vi "fgv_file_data.vi"(7 "cmd_file":T1(ring), 8 "err in":errorcluster caption="에러 입력(에러 없음)") -> (0 "error out":errorcluster, 1 "Fail event table":string[][](table), 2 "Strain":waveform(dbl)[](array[waveform]), 3 "Res Acc":waveform(dbl)[](array[waveform]))   [LabVIEW 2016]
panel:
  in  "file path":path
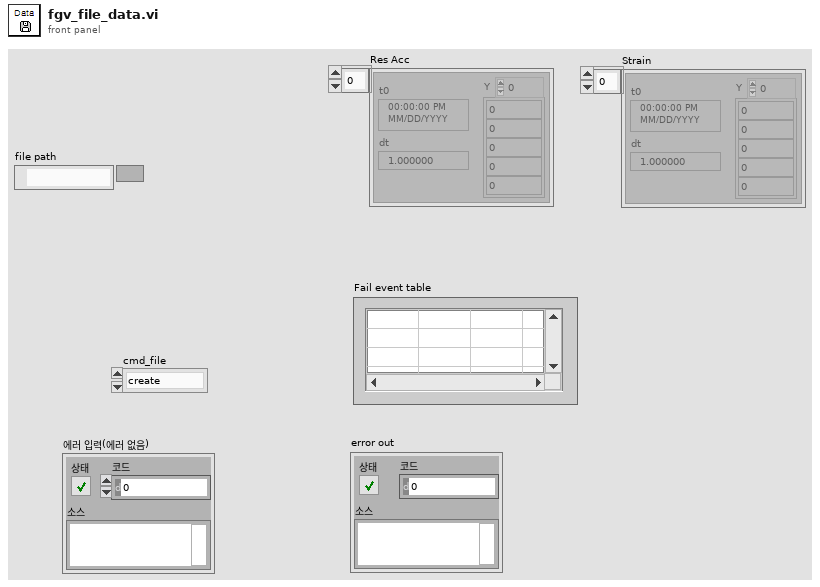
[diagram p1: front panel]
types:
  T1 = enum16{"create", "write_data", "write_event", "read_data", "read_event", "close"}
  T2 = typedef "Total data.ctl" = cluster{"Raw Data":T3, "Resister result data":T4, "Result Table update":cluster{"Num":u32[], "Resister 1~5":u8[][], "Resister 6~10":u8[][], "Resister 11~15":u8[][]}, "Strain Data":cluster{"Strain 1":dbl, "Strain 2":dbl, "Strain 3":dbl, "Strain 4":dbl}, "Acc Result":cluster{"Acc Peak":dbl, "Acc time":dbl, "Acc area":dbl}, "STATUS":cluster{"status":string, "all_fail":bool, "emg":bool, "cycle":u16, "file name":string}, "Speed":dbl, "Acc peak time":dbl, "Max Strain":dbl, "Resistor at peak":cluster{"[0]":dbl, "[1]":dbl, "[2]":dbl, "[3]":dbl, "[4]":dbl, "[5]":dbl, "[6]":dbl, "[7]":dbl, "[8]":dbl, "[9]":dbl, "[10]":dbl, "[11]":dbl, "[12]":dbl, "[13]":dbl, "[14]":dbl}, "Acc peak index":u32, "time":string, "Cycle finish":bool, "Resistor at ini":cluster{"[0]":dbl, "[1]":dbl, "[2]":dbl, "[3]":dbl, "[4]":dbl, "[5]":dbl, "[6]":dbl, "[7]":dbl, "[8]":dbl, "[9]":dbl, "[10]":dbl, "[11]":dbl, "[12]":dbl, "[13]":dbl, "[14]":dbl}}
  T3 = typedef "raw Q data.ctl" = cluster{"Res_data":waveform(dbl)[], "Acc_data":waveform(dbl), "Strain_data":waveform(dbl)[]}
  T4 = typedef "raw data type.ctl" = cluster{"Resistor values":cluster{"[0]":dbl, "[1]":dbl, "[2]":dbl, "[3]":dbl, "[4]":dbl, "[5]":dbl, "[6]":dbl, "[7]":dbl, "[8]":dbl, "[9]":dbl, "[10]":dbl, "[11]":dbl, "[12]":dbl, "[13]":dbl, "[14]":dbl}, "Resistor tables":u8[], "Pass Fails":bool[]}
  T5 = cluster{"Test Information":cluster{"date":string, "custom":string, "oper":string, "package":string, "pkg side":string, "solder":string, "brd side":string, "paste":string, "reflow":string}, "Sensor Set":cluster{"Accelerometer":cluster{"Sensitivity(mV/g)":dbl}, "Strain Guage":cluster{"Ch.":dbl[], "Gage factor":dbl[], "Resistance":dbl[], "Poisson ratio":dbl[]}}, "Resistor Set":cluster{"Criterion Level":dbl, "Res. Set":cluster{"Res. Ch":dbl, "Res. Active":bool, "Res Initial":dbl}[]}, "Test Stop Condition":cluster{"Test cycle":u16, "Fail number in a cycle":u16, "Fail factor":cluster{"Duration":u16, "Fail No.":u16}}, "Acceleration Condition ":cluster{"Shock duration pecent [%]":u16, "Filter cutoff freq":u32}, "Save":cluster{"Save Path":path, "File Name":string}}
  T6 = enum16{"open", "open or create", "create or replace", "create", "open (read-only)"}
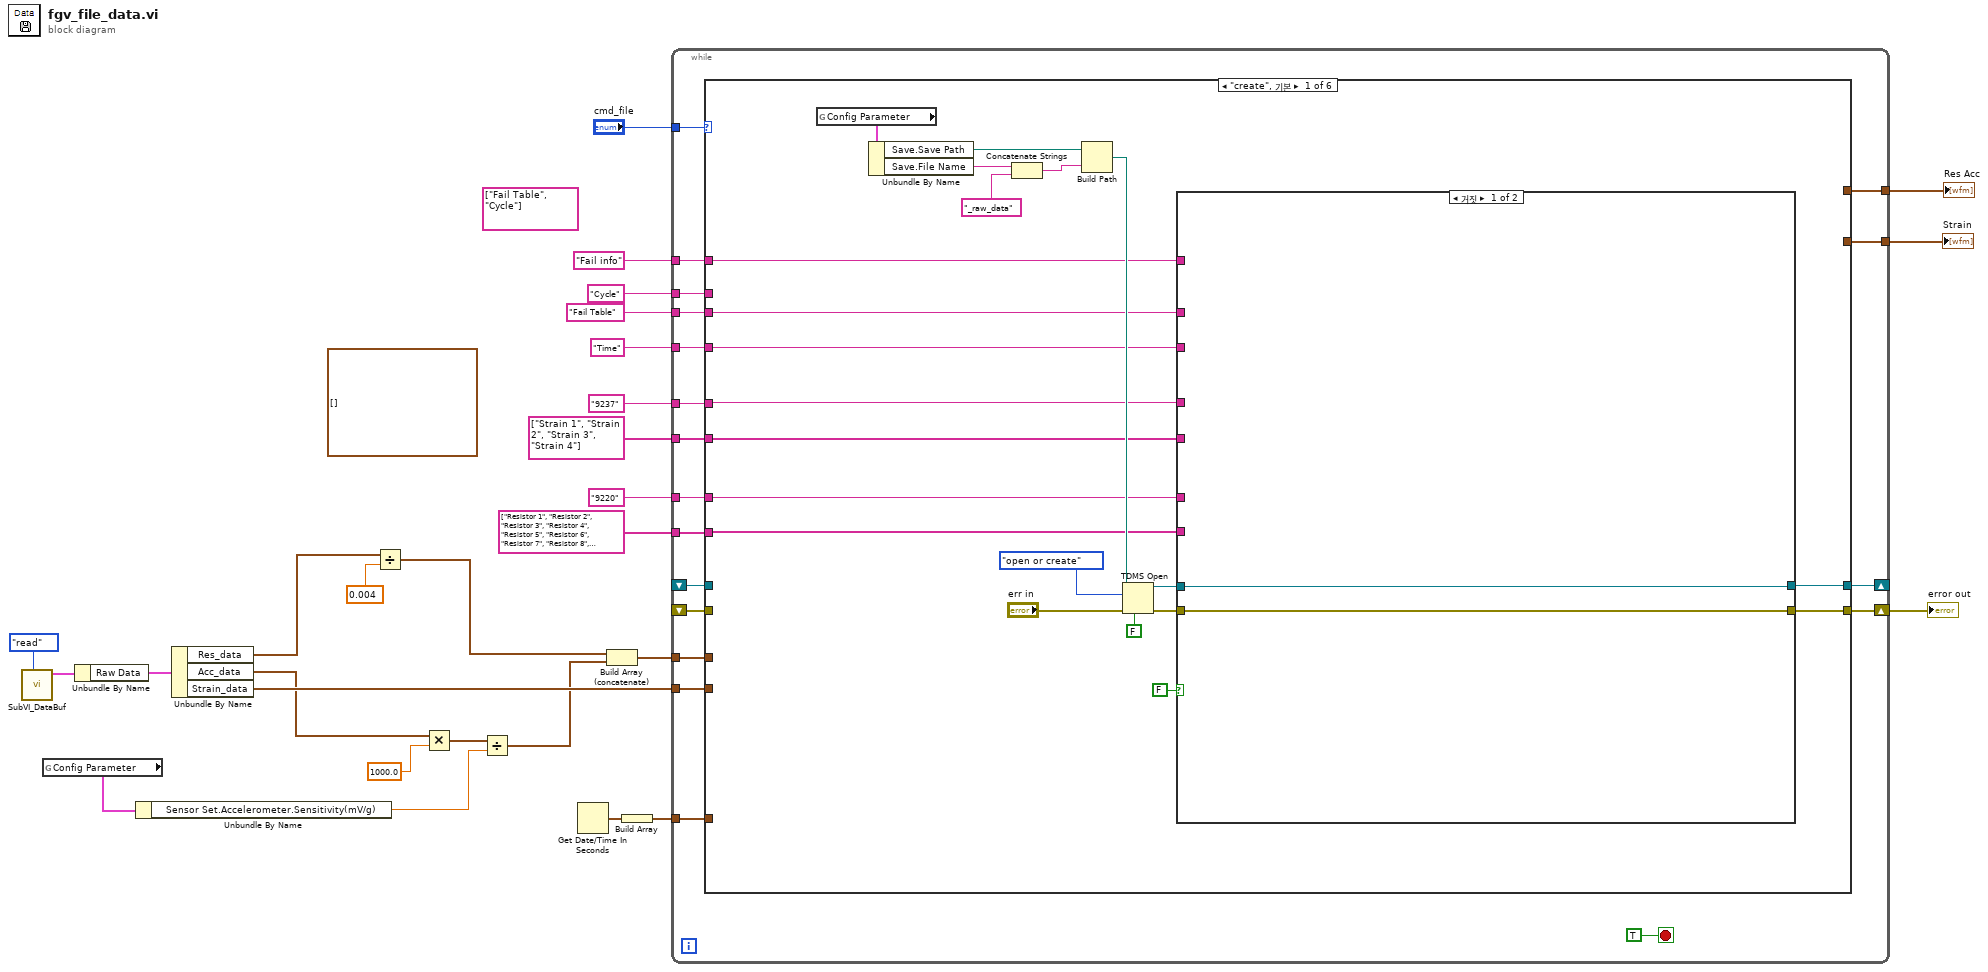
[diagram p0: block diagram]
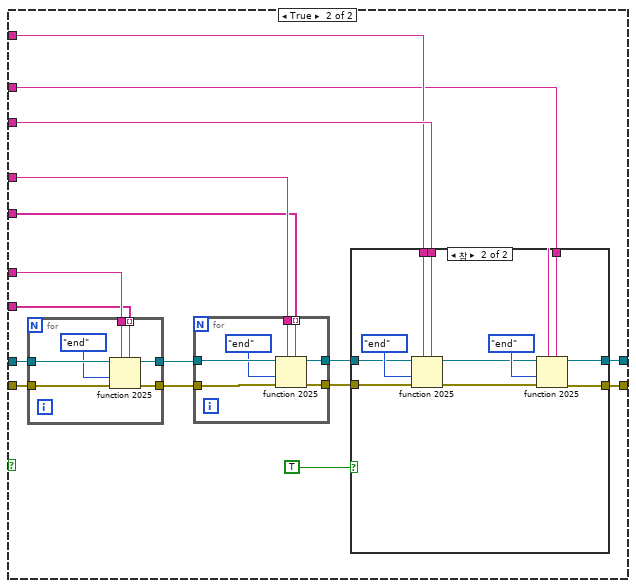
[diagram p2: hidden frame]
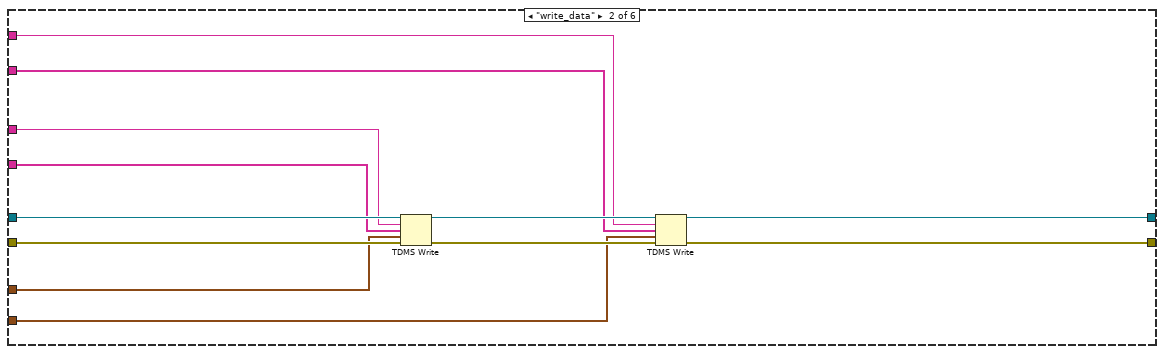
[diagram p4: hidden frame]
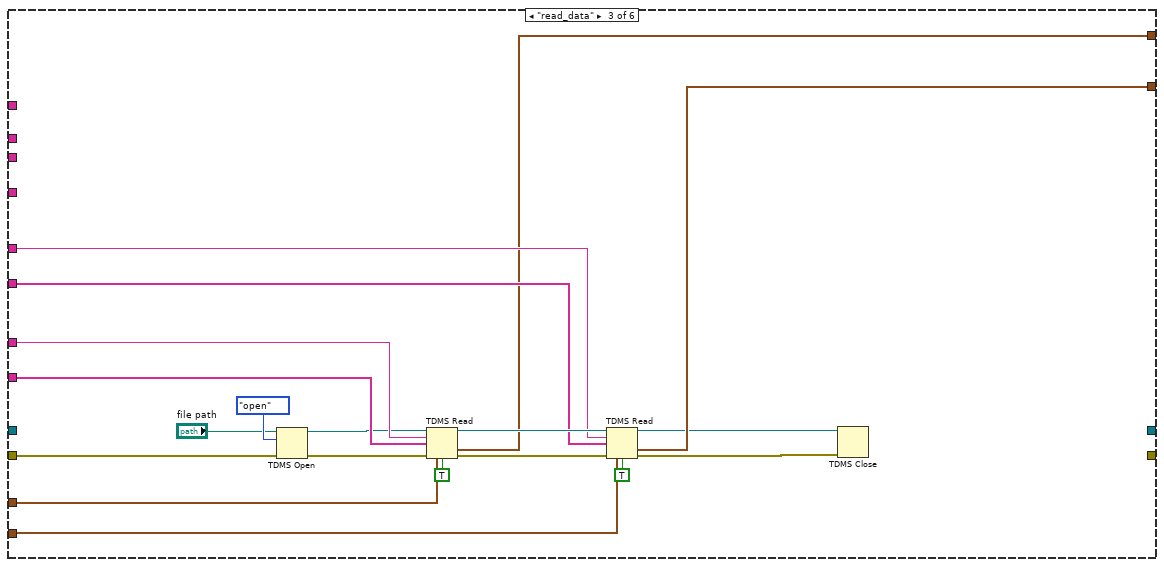
[diagram p5: hidden frame]
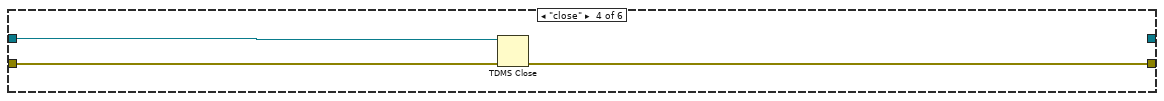
[diagram p6: hidden frame]
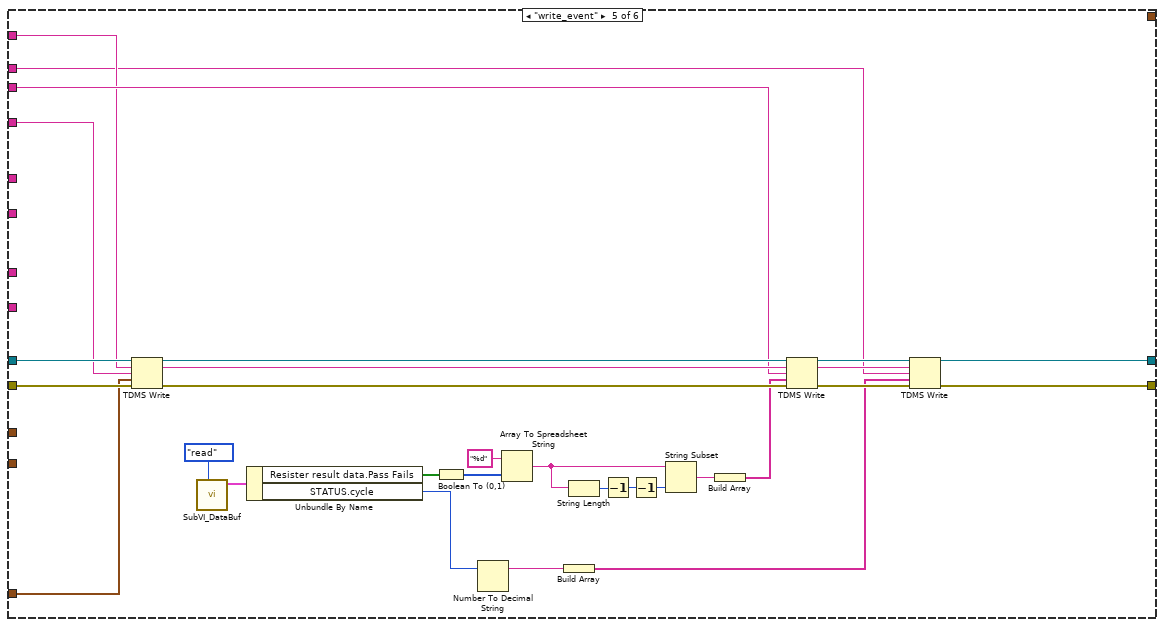
[diagram p7: hidden frame]
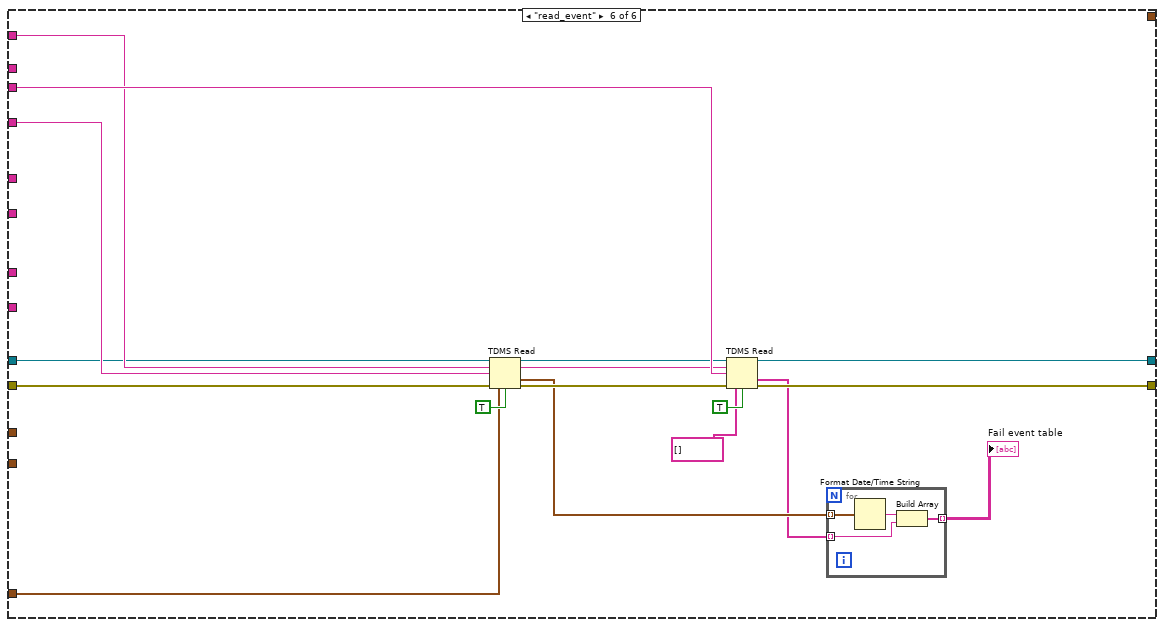
[diagram p8: hidden frame]
diagram:
  (unwired) string[] ["Fail Table", "Cycle"]
  (unwired) waveform(dbl)[] [] ("Strain_data")
  n1 = call "SubVI_DataBuf.vi"("cmd"=enum16{"ini", "write", "read"}."read") -> ("Total data 2"=w19:T2)  [unwired: 9 in, 1 out]
  n2 = global read "글로벌_Config Parameter.vi" "Config Parameter"() -> (w3:T5)
  n3 = Unbundle By Name(w19) -> ("Raw Data"=w20:T3)
  n4 = Unbundle By Name(w3) -> ("Sensor Set.Accelerometer.Sensitivity(mV/g)"=w6:dbl)
  n5 = Unbundle By Name(w20) -> ("Res_data"=w10:waveform(dbl)[], "Acc_data"=w5:waveform(dbl), "Strain_data"=w16:waveform(dbl)[])
  n6 = Divide(x=w10, y=0.004) -> (x/y=w9:waveform(dbl)[])
  n7 = Multiply(x=w5, y=1000.0) -> (x*y=w7:waveform(dbl))
  n8 = Divide(x=w7, y=w6) -> (x/y=w4:waveform(dbl))
  n9 = Get Date/Time In Seconds() -> (seconds since 1Jan1904=w22:timestamp)
  n10 = Build Array (concatenate)(w9, w4) -> (w17:waveform(dbl)[])
  n11 = Build Array(w22) -> (w21:timestamp[])
  n12 = while {
    shift-right: [w45] -> _
    shift-left: _ -> [w44]
    shift-right: [w42] -> w27
    shift-left: _ -> [w43]
    tunnel: "cmd_file" -> [w46]
    tunnel: string[] ["Resistor 1", "Resistor 2", "Resistor 3", "Resistor 4", "Resistor 5", "Resistor 6", "Resistor 7", "Resistor 8", "Resistor 9", "Resistor 10", "Resistor 11", "Resistor 12", "Resistor 13", "Resistor 14", "Resistor 15", "Acc"] ("채널 이름 입력(제목없음)") -> [w41]
    tunnel: "9220" ("그룹 이름 입력(제목없음)") -> [w40]
    tunnel: "9237" ("그룹 이름 입력(제목없음)") -> [w39]
    tunnel: string[] ["Strain 1", "Strain 2", "Strain 3", "Strain 4"] ("채널 이름 입력(제목없음)") -> [w38]
    tunnel: w21 -> [w37]
    tunnel: w17 -> [w36]
    tunnel: w16 -> [w35]
    tunnel: "Fail Table" ("channel name") -> [w34]
    tunnel: "Fail info" ("group name") -> [w33]
    tunnel: "Time" ("channel name") -> [w32]
    tunnel: "Cycle" ("channel name") -> [w31]
    tunnel: [w30] -> w2
    tunnel: [w29] -> w1
    stop <- TRUE stop-if-true
    n13 = case shown="\"create\", 기본" w46 {
      tunnel: [w49 w120 _ _ w153 w187] -> w45
      tunnel: w44 -> [_ w124 _ w147 w173 w179]
      tunnel: w43 -> [_ w125 w131 w146 w172 w189]
      tunnel: [w51 w121 _ w145 w152 w188] -> w42
      tunnel: w41 -> [w58 w119 w142 _ _ _]
      tunnel: w40 -> [w59 w118 w143 _ _ _]
      tunnel: w39 -> [w57 w117 w137 _ _ _]
      tunnel: w38 -> [w56 w116 w136 _ _ _]
      tunnel: w37 -> [_ _ _ _ w169 w185]
      tunnel: w36 -> [_ w115 w141 _ _ _]
      tunnel: w35 -> [_ w114 w135 _ _ _]
      tunnel: w34 -> [w53 _ _ _ w159 w190]
      tunnel: w33 -> [w54 _ _ _ w158 w181]
      tunnel: w32 -> [w55 _ _ _ w157 w180]
      tunnel: w31 -> [_ _ _ _ w150 _]
      tunnel: [_ _ w134 _ _ _] -> w30
      tunnel: [_ _ w133 _ _ _] -> w29
      frame "create", Default {
        n14 = global read "글로벌_Config Parameter.vi" "Config Parameter"() -> (w65:T5)
        n15 = Unbundle By Name(w65) -> ("Save.Save Path"=w64:path, "Save.File Name"=w61:string)
        n16 = Concatenate Strings(w61, "_raw_data" ("문자열")) -> (w60:string)
        n17 = Build Path(base path=w64, name or relative path=w60) -> (appended path=w63:path)
        n18 = TDMS Open(6:FALSE ("disable buffering (T)"), 8:"err in", 10:T6."open or create" ("operation"), 11:w63) -> (0:w52:errorcluster, 3:w50:refnum<k34>)  [unwired: 3 in]
        n19 = case shown="거짓" FALSE {
          tunnel: w59 -> [_ w86]
          tunnel: w58 -> [_ w85]
          tunnel: w57 -> [_ w82]
          tunnel: w56 -> [_ w81]
          tunnel: w55 -> [_ w78]
          tunnel: w54 -> [_ w77]
          tunnel: w53 -> [_ w76]
          tunnel: w52 -> [w69 w75]
          tunnel: [w69 w74] -> w51
          tunnel: w50 -> [w70 w73]
          tunnel: [w70 w72] -> w49
          frame False {
          }
          frame True {
            n20 = for {
              tunnel: w73 -> [w113]
              tunnel: w75 -> [w112]
              tunnel: w86 -> [w110]
              tunnel: w85 -> [w109] mode=indexing
              tunnel: [w108] -> w84
              tunnel: [w107] -> w83
              n21 = fn#2025(5:w109, 7:w110, 8:w112, 9:enum16{"start", "end"}."end" ("시작(0:시작)"), 11:w113) -> (0:w107:errorcluster, 3:w108:refnum<k34>)  [unwired: 1 in]
            }
            n22 = for {
              tunnel: w84 -> [w106]
              tunnel: w83 -> [w105]
              tunnel: w82 -> [w103]
              tunnel: w81 -> [w102] mode=indexing
              tunnel: [w101] -> w80
              tunnel: [w100] -> w79
              n23 = fn#2025(5:w102, 7:w103, 8:w105, 9:enum16{"start", "end"}."end" ("시작(0:시작)"), 11:w106) -> (0:w100:errorcluster, 3:w101:refnum<k34>)  [unwired: 1 in]
            }
            n24 = case shown="참" TRUE {
              tunnel: w80 -> [w88 w98]
              tunnel: w79 -> [w87 w97]
              tunnel: w78 -> [_ w96]
              tunnel: w77 -> [_ w93]
              tunnel: w76 -> [_ w92]
              tunnel: [w87 w90] -> w74
              tunnel: [w88 w89] -> w72
              frame False {
              }
              frame True {
                n25 = fn#2025(5:w96, 7:w93, 8:w97, 9:enum16{"start", "end"}."end" ("시작(0:시작)"), 11:w98) -> (0:w95:errorcluster, 3:w91:refnum<k34>)  [unwired: 1 in]
                n26 = fn#2025(5:w92, 7:w93, 8:w95, 9:enum16{"start", "end"}."end" ("시작(0:시작)"), 11:w91) -> (0:w90:errorcluster, 3:w89:refnum<k34>)  [unwired: 1 in]
              }
            }
          }
        }
      }
      frame "write_data" {
        n27 = TDMS Write(0:w124, 5:w118, 7:w119, 9:w115, 11:w125) -> (4:w122:refnum<k34>, 15:w123:errorcluster)  [unwired: 1 in, 2 out]
        n28 = TDMS Write(0:w122, 5:w117, 7:w116, 9:w114, 11:w123) -> (4:w120:refnum<k34>, 15:w121:errorcluster)  [unwired: 1 in, 2 out]
      }
      frame "read_data" {
        n29 = TDMS Open(8:w131, 10:T6."open" ("operation"), 11:"file path") -> (0:w130:errorcluster, 3:w128:refnum<k34>)  [unwired: 4 in]
        n30 = TDMS Read(0:w128, 5:w143, 7:w142, 11:w130, 12:w141, 13:TRUE ("return channels in file order? (F)")) -> (4:w139:refnum<k34>, 10:w134:waveform(dbl)[], 15:w140:errorcluster)  [unwired: 2 in, 3 out]
        n31 = TDMS Read(0:w139, 5:w137, 7:w136, 11:w140, 12:w135, 13:TRUE ("return channels in file order? (F)")) -> (4:w126:refnum<k34>, 10:w133:waveform(dbl)[], 15:w127:errorcluster)  [unwired: 2 in, 3 out]
        n32 = TDMS Close(8:w127, 11:w126) -> ()  [unwired: 2 out]
      }
      frame "close" {
        n33 = TDMS Close(8:w146, 11:w147) -> (0:w145:errorcluster)  [unwired: 1 out]
      }
      frame "write_event" {
        n34 = TDMS Write(0:w173, 5:w158, 7:w157, 9:w169, 11:w172) -> (4:w175:refnum<k34>, 6:w176:string, 15:w174:errorcluster)  [unwired: 1 in, 1 out]
        n35 = call "SubVI_DataBuf.vi"("cmd"=enum16{"ini", "write", "read"}."read") -> ("Total data 2"=w170:T2)  [unwired: 9 in, 1 out]
        n36 = Unbundle By Name(w170) -> ("Resister result data.Pass Fails"=w162:bool[], "STATUS.cycle"=w148:u16)
        n37 = Boolean To (0,1)(Boolean=w162) -> (0, 1=w168:i16[])
        n38 = Number To Decimal String(number=w148) -> (decimal integer string=w149:string)  [unwired: 1 in]
        n39 = Array To Spreadsheet String(array=w168, 3:"%d" ("포맷 문자열")) -> (spreadsheet string=w166:string)  [unwired: 1 in]
        n40 = Build Array(w149) -> (w151:string[])
        n41 = String Length(string=w166) -> (length=w165:i32)
        n42 = Decrement(x=w165) -> (x-1=w164:i32)
        n43 = Decrement(x=w164) -> (x-1=w163:i32)
        n44 = String Subset(string=w166, length (rest)=w163) -> (substring=w161:string)  [unwired: 1 in]
        n45 = Build Array(w161) -> (w160:string[])
        n46 = TDMS Write(0:w175, 5:w176, 7:w159, 9:w160, 11:w174) -> (4:w155:refnum<k34>, 6:w156:string, 15:w154:errorcluster)  [unwired: 1 in, 1 out]
        n47 = TDMS Write(0:w155, 5:w156, 7:w150, 9:w151, 11:w154) -> (4:w153:refnum<k34>, 15:w152:errorcluster)  [unwired: 1 in, 2 out]
      }
      frame "read_event" {
        n48 = TDMS Read(0:w179, 5:w181, 7:w180, 12:w185, 13:TRUE ("return channels in file order? (F)")) -> (4:w178:refnum<k34>, 6:w184:string, 10:w183:timestamp[])  [unwired: 3 in, 3 out]
        n49 = TDMS Read(0:w178, 5:w184, 7:w190, 11:w189, 12:string[] [], 13:TRUE ("return channels in file order? (F)")) -> (4:w187:refnum<k34>, 10:w182:string[], 15:w188:errorcluster)  [unwired: 2 in, 3 out]
        n50 = for {
          tunnel: w183 -> [w196] mode=indexing
          tunnel: w182 -> [w194] mode=indexing
          tunnel: [w193] -> w177 mode=indexing
          n51 = Format Date/Time String(seconds (now)=w196) -> (date/time string=w195:string)  [unwired: 2 out]
          n52 = Build Array(w195, w194) -> (w193:string[])
        }
        "Fail event table" <- w177
      }
    }
  }
  "error out" <- w27
  "Res Acc" <- w2
  "Strain" <- w1
